vi "Post-Install Update Alert.vi"() -> ()   [LabVIEW 2020]
panel:
  in  "OK":bool
  # "If you've already started a project and have just updated the SquareBattle project, be sure to pull in the changes with the project updater in the Tools -> Summer of LabVIEW menu entry from your existing project. This will pull in any bugfixes, new teams to test against, and will automatically update your team code to maintain compatibility with engine changes."
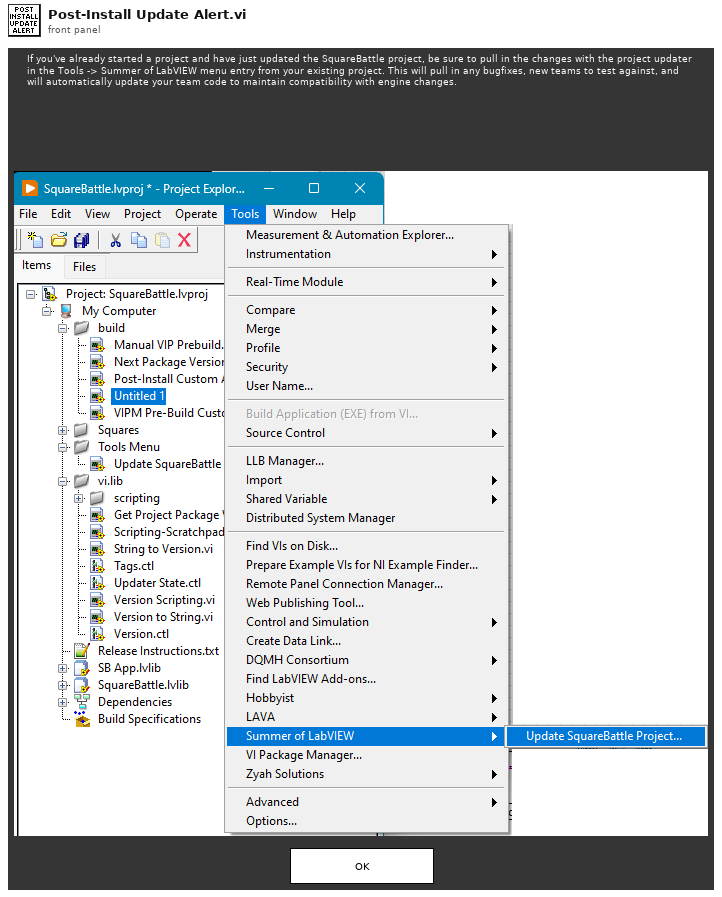
[diagram p1: front panel]
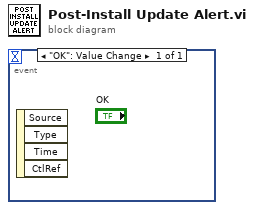
[diagram p0: block diagram]
diagram:
  n1 = event shown="[0] \"OK\": Value Change" {
    selector: _ -> [_]
    dyn-events: _ -> [_]
    timeout: _ -> [_]
    event "OK": Value Change {
      n2 = event-data() -> ()  [unwired: 1 in, 4 out]
    }
  }
